vi "AFG3352X.set output mode.vi"(0 "i ref in":refnum<vi>, 1 "Channel (1: 1)":i32(ring)=1 items=["1"=1, "2"=2], 2 "Output State (0: Normal)":i32(ring) items=["Normal", "Gated"], 3 "ms timeout (10000)":i32=10000, 5 "error in (no error)":errorcluster) -> (14 "i ref out":refnum<vi>, 17 "timed out":bool, 19 "error out":errorcluster)   [LabVIEW 2014, in "AFG3352X.lvlib"]
doc: "Sets the frequency at my device."
uses:
  AFG3352X.lvlib
  CSCore/CSApplicationBaseClasses/AFGBase/AFGBase.directionType.ctl
  CSlibraries/UtilityLib/UtilityLib.valueStatus.ctl
  CSCore/CSApplicationBaseClasses/DeviceBase/DeviceBase.lvlib
  CSCore/CSApplicationBaseClasses/AFGBase/AFGBase.lvlib
  CSlibraries/UtilityLib/UtilityLib.lvlib
  CSinstr.lib/Agilent 3352X Series/Agilent 3352X Series.lvlib
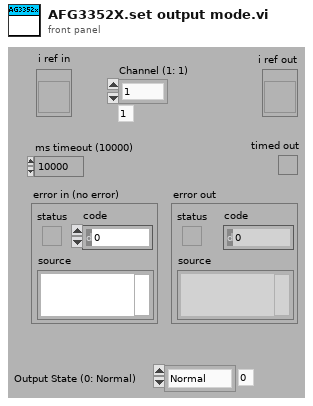
[diagram p1: front panel]
types:
  T1 = typedef "UtilityLib.lvlib/UtilityLib.valueStatus.ctl" = enum16{"no info available", "stand by/off", "on", "warning", "alarm/malfunction", "not implemented", "user action required", "important information", "system default", "control default", "indicator default", "button default"}
  T2 = typedef "AFGBase.lvlib/AFGBase.directionType.ctl" = enum16{"unknown", "update actual value", "update nominal value", "update both"}
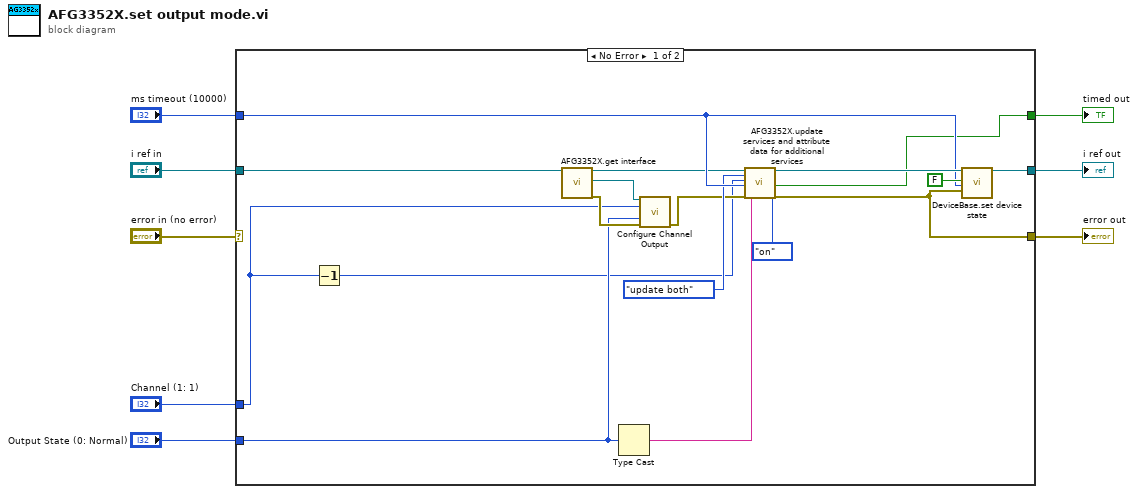
[diagram p0: block diagram]
diagram:
  n1 = case shown="No Error" "error in (no error)" {
    selector: "error in (no error)" -> [_ w26]
    tunnel: [w25 w27] -> w8
    tunnel: "ms timeout (10000)" -> [w21 _]
    tunnel: "i ref in" -> [w11 w27]
    tunnel: [w22 w26] -> w4
    tunnel: "Output State (0: Normal)" -> [w13 _]
    tunnel: [w17 _] -> w3
    tunnel: "Channel (1: 1)" -> [w10 _]
    frame No Error {
      n2 = Decrement(x=w10) -> (x-1=w9:i32)
      n3 = call "AFG3352X.get interface.vi"("i ref in"=w11) -> ("i ref out"=w18:refnum<vi>, "interface"=w16:refnum<visa-resource-name>, "error out"=w15:errorcluster)  [unwired: 16 in]
      n4 = Type Cast(x=w13) -> (*(type *) &x=w20:string)  [unwired: 1 in]
      n5 = call "Configure Channel Output.vi"("VISA resource name"=w16, "Channel (1: 1)"=w10, "Output State (0: Normal)"=w13, "error in (no error)"=w15) -> ("error out"=w14:errorcluster)  [unwired: 10 in, 1 out]
      n6 = call "AFG3352X.update services and attribute data for additional services.vi"("i ref in"=w18, "direction"=AFGBase.directionType."update both", "Service"=w9, "ms timeout (10000)"=w21, "value"=w20, "error in (no error)"=w14, "quality"=UtilityLib.valueStatus."on") -> ("i ref out"=w23:refnum<vi>, "timed out"=w17:bool, "error out"=w22:errorcluster)  [unwired: 10 in]
      n7 = call "DeviceBase.set device state.vi"("i ref in"=w23, "implicit"=FALSE, "ms timeout (10000)"=w21, "device error"=w22) -> ("i ref out"=w25:refnum<vi>)  [unwired: 13 in, 2 out]
    }
    frame Error {
    }
  }
  "error out" <- w4
  "i ref out" <- w8
  "timed out" <- w3
